vi "laboratorio_07_Ivan.vi"() -> ()   [LabVIEW 2024]
uses:
  <vilib>/Utility/error.llb/Trim Whitespace One-Sided.vi
  <vilib>/Instr/_visa.llb/VISA Configure Serial Port (Instr).vi
  <vilib>/Analysis/NI_AALPro.lvlib
panel:
  out "error out 1":errorcluster
  out "error out 2":errorcluster
  out "error out 3":errorcluster
  out "Segnale":cluster{"Best Exponential Fit":dbl[], dbl[]}[](graph)
  out "ADC NL":cluster{dbl[], dbl[]}(graph)
  out "Residui":cluster{dbl[], dbl[]}(graph)
  out "offset":dbl
  out "C(pF)":dbl
  in  "Medie":bool
  in  "dt":dbl
  in  "stop":bool
  in  "length":i32
  in  "begin":i32
  in  "VISA resource name":refnum<visa-resource-name>
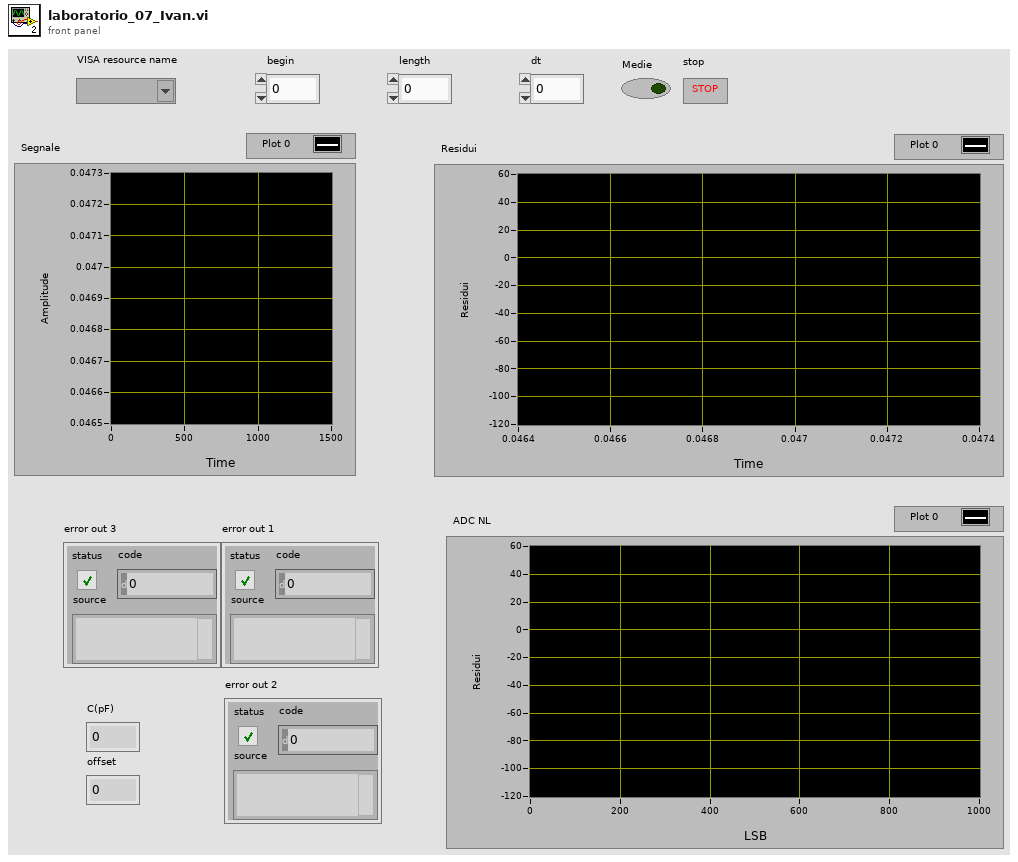
[diagram p1: front panel]
types:
  T1 = enum16{"open", "replace", "create", "open or create", "replace or create", "replace or create with confirmation"}
  T2 = cluster{"amp min":dbl, "amp max":dbl, "damping min":dbl, "damping max":dbl, "offset min":dbl, "offset max":dbl}
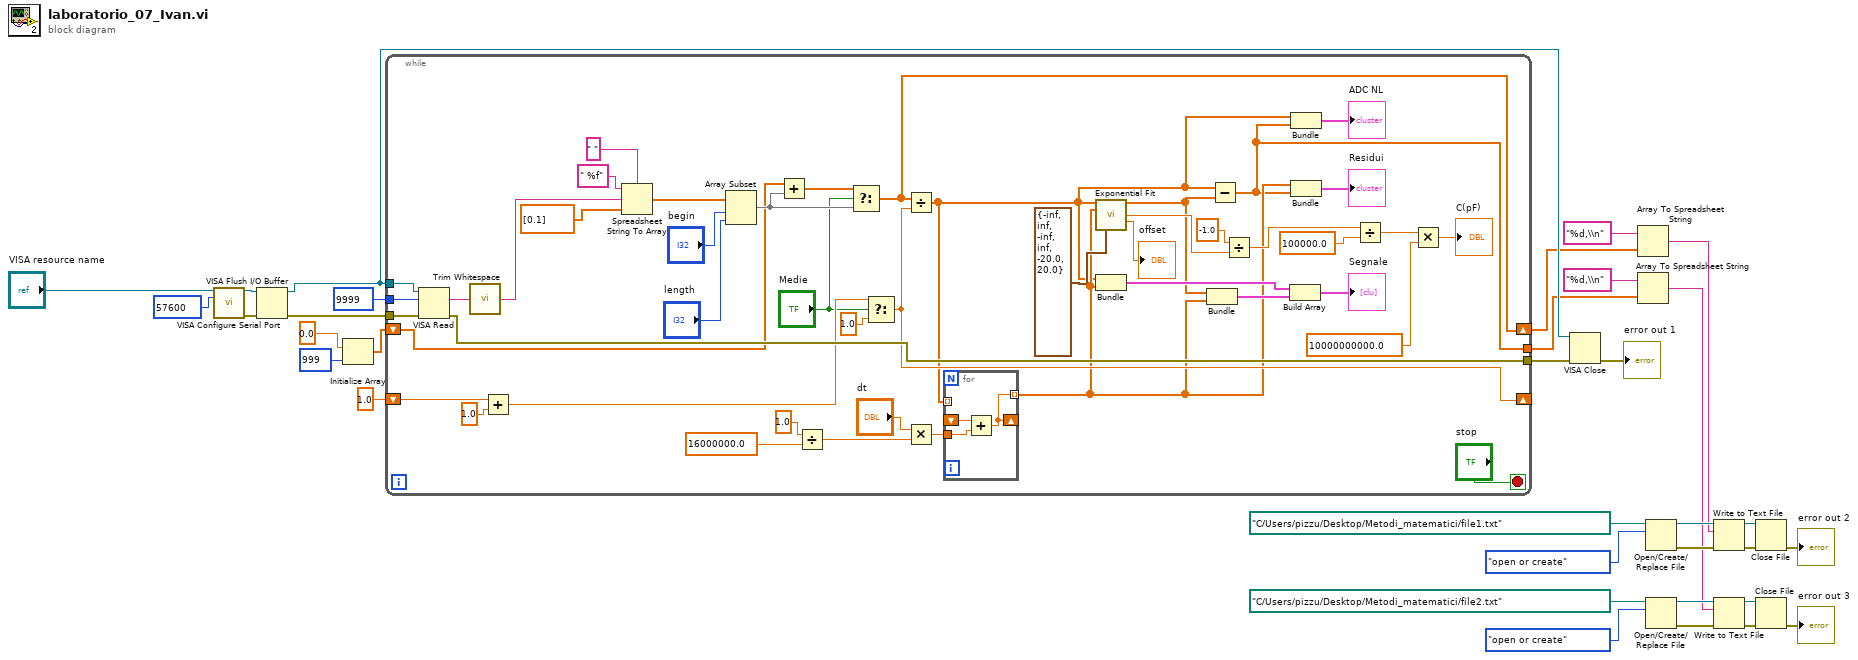
[diagram p0: block diagram]
diagram:
  n1 = call-poly "VISA Configure Serial Port"("VISA resource name"="VISA resource name", "baud rate (9600)"=u32 57600) -> ("VISA resource name out"=w31:refnum<visa-resource-name>, "error out"=w30:errorcluster)  [unwired: 12 in]
  n2 = VISA Flush I/O Buffer(VISA resource name=w31, error in (no error)=w30) -> (VISA resource name out=w26:refnum<visa-resource-name>, error out=w29:errorcluster)  [unwired: 1 in]
  n3 = Initialize Array(0.0 ("element"), 999 ("dimension size")) -> (w3:dbl[])
  n4 = while {
    tunnel: w29 -> [w79]
    tunnel: w26 -> [w78]
    tunnel: u32 9999 ("byte count") -> [w77]
    tunnel: [w68] -> w27
    shift-right: [w50] -> _
    shift-left: 1.0 ("x") -> [w51]
    tunnel: [w37] -> w5
    shift-right: [w35] -> w2
    shift-left: w3 -> [w36]
    stop <- "stop" stop-if-true
    n5 = VISA Read(VISA resource name=w78, byte count=w77, error in (no error)=w79) -> (read buffer=w76:string, error out=w68:errorcluster)  [unwired: 2 out]
    n6 = call <vilib>:"Trim Whitespace.vi"("string"=w76) -> ("trimmed string"=w75:string)  [unwired: 1 in]
    n7 = Add(x=w51, y=1.0) -> (x+y=w67:dbl)
    n8 = Spreadsheet String To Array(delimiter (Tab)=" ", format string=" %f", spreadsheet string=w75, array type (2D Dbl)=dbl[] [0.1]) -> (array=w71:dbl[])
    n9 = Array Subset(array=w71, index="begin", length="length") -> (w58:dbl[])
    n10 = Add(x=w36, y=w58) -> (x+y=w59:dbl[])
    n11 = Divide(x=1.0, y=16000000.0) -> (x/y=w63:dbl)
    n12 = Select(t=w59, s="Medie", f=w58) -> (s? t:f=w35:dbl[])
    n13 = Select(t=w67, s="Medie", f=1.0) -> (s? t:f=w50:dbl)
    n14 = Divide(x=w35, y=w50) -> (x/y=w42:dbl[])
    n15 = Multiply(x="dt", y=w63) -> (x*y=w49:dbl)
    n16 = for {
      tunnel: w42 -> [_] mode=indexing
      shift-right: [w80] -> _
      shift-left: _ -> [w82]
      tunnel: w49 -> [w81]
      tunnel: [w80] -> w43 mode=indexing
      n17 = Add(x=w82, y=w81) -> (x+y=w80:dbl)
    }
    n18 = call <vilib>:"Exponential Fit.vi"("Y"=w42, "X"=w43, "parameter bounds"=T2 {"amp min"=-inf, "amp max"=inf, "damping min"=-inf, "damping max"=inf, "offset min"=-20.0, "offset max"=20.0}) -> ("Best Exponential Fit"=w41:dbl[], "damping"=w47:dbl, "offset"=→"offset":dbl)  [unwired: 7 in, 3 out]
    n19 = Bundle(w42, w43) -> (w45:cluster{dbl[], dbl[]})  [unwired: 1 in]
    n20 = Bundle("Best Exponential Fit"=w41, w43) -> (w44:cluster{"Best Exponential Fit":dbl[], dbl[]})  [unwired: 1 in]
    n21 = Subtract(x=w42, y=w41) -> (x-y=w37:dbl[])
    n22 = Divide(x=-1.0, y=w47) -> (x/y=w56:dbl)
    n23 = Build Array(w45, w44) -> (→"Segnale":cluster{"Best Exponential Fit":dbl[], dbl[]}[])
    n24 = Bundle(w42, w37) -> (→"ADC NL":cluster{dbl[], dbl[]})  [unwired: 1 in]
    n25 = Bundle(w43, w37) -> (→"Residui":cluster{dbl[], dbl[]})  [unwired: 1 in]
    n26 = Divide(x=w56, y=100000.0) -> (x/y=w53:dbl)
    n27 = Multiply(x=w53, y=10000000000.0) -> (x*y=→"C(pF)":dbl)
  }
  n28 = VISA Close(VISA resource name=w26, error in (no error)=w27) -> (error out=→"error out 1":errorcluster)
  n29 = Array To Spreadsheet String(array=w2, 3:"%d,\\n" ("format string")) -> (spreadsheet string=w1:string)  [unwired: 1 in]
  n30 = Array To Spreadsheet String(array=w5, 3:"%d,\\n" ("format string")) -> (spreadsheet string=w4:string)  [unwired: 1 in]
  n31 = Open/Create/Replace File(file path (use dialog)=path "C:/Users/pizzu/Desktop/Metodi_matematici/file1.txt", operation (0:open)=T1."open or create") -> (refnum out=w22:refnum<file>, error out=w14:errorcluster)  [unwired: 4 in, 1 out]
  n32 = Open/Create/Replace File(file path (use dialog)=path "C:/Users/pizzu/Desktop/Metodi_matematici/file2.txt", operation (0:open)=T1."open or create") -> (refnum out=w20:refnum<file>, error out=w12:errorcluster)  [unwired: 4 in, 1 out]
  n33 = Write to Text File(file (use dialog)=w22, text=w1, error in=w14) -> (refnum out=w21:refnum<file>, error out=w13:errorcluster)  [unwired: 1 in, 1 out]
  n34 = Write to Text File(file (use dialog)=w20, text=w4, error in=w12) -> (refnum out=w19:refnum<file>, error out=w11:errorcluster)  [unwired: 1 in, 1 out]
  n35 = Close File(refnum=w21, error in=w13) -> (error out=→"error out 2":errorcluster)  [unwired: 1 out]
  n36 = Close File(refnum=w19, error in=w11) -> (error out=→"error out 3":errorcluster)  [unwired: 1 out]
